vi "Read Size.vi"(8 "error in (no error)":errorcluster, 11 "Splitter in":refnum<class "Splitter.lvclass">) -> (0 "error out":errorcluster, 2 "Size":i32, 3 "Splitter out":refnum<class "Splitter.lvclass">)   [LabVIEW 2017, in "Splitter.lvclass"]
uses:
  Splitter.lvclass
  Splitter.lvclass/Splitter.ctl
  Low-Level VI Manipulation/Find Resource by Type (String).vi
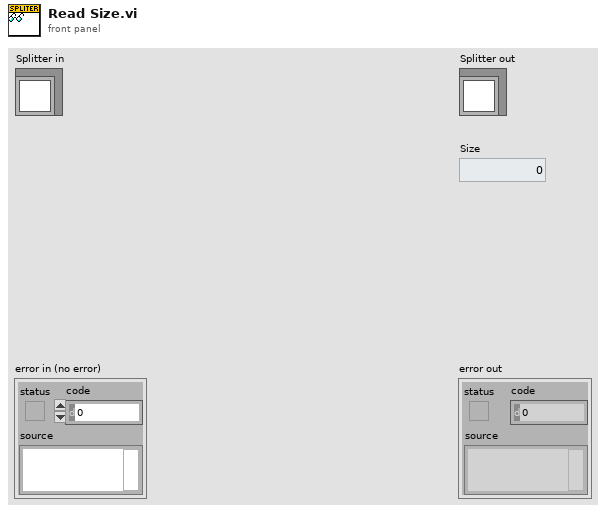
[diagram p1: front panel]
types:
  T1 = typedef "Resource Array.ctl" = T2[]
  T2 = typedef "Resource.ctl" = cluster{"type":u32, "id":i32, "name":string, "binary data":string}
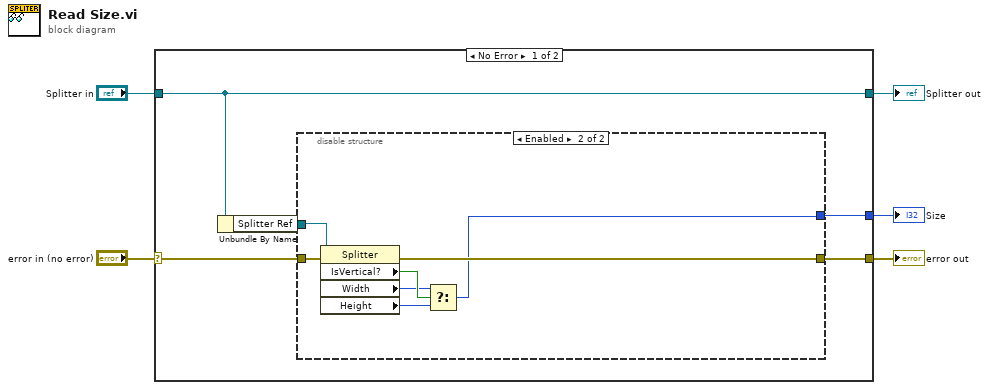
[diagram p0: block diagram]
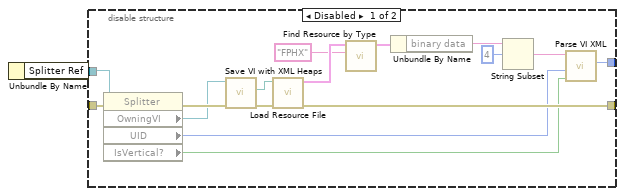
[diagram p2: hidden frame]
diagram:
  n1 = case shown="No Error" "error in (no error)" {
    selector: "error in (no error)" -> [w8 w35]
    tunnel: [w7 w35] -> w4
    tunnel: [w9 w36] -> w2
    tunnel: "Splitter in" -> [w9 w36]
    tunnel: [w6 _] -> w1
    frame No Error {
      n2 = disable-structure shown="Enabled" {
        disable-tunnel: w9 -> [w26 w34]
        disable-tunnel: w8 -> [w18 w33]
        disable-tunnel: [w17 w31] -> w7
        disable-tunnel: [w12 w27] -> w6
        frame Disabled {
          n3 = Unbundle By Name(w26) -> ("Splitter Ref"=w11:refnum<vi>)
          n4 = property class="Splitter"(reference=w11, error in=w18) -> (error out=w15:errorcluster, "OwningVI"=w10:refnum<vi>, "UID"=w14:i32, "IsVertical?"=w13:bool)  [unwired: 1 out]
          n5 = call "Save VI with XML Heaps.vi"("error in (no error)"=w15, "VI Refnum In"=w10) -> ("error out"=w19:errorcluster, "VI Path out"=w25:path)  [unwired: 7 in, 1 out]
          n6 = call "Load Resource File.vi"("error in (no error)"=w19, "Resource file"=w25) -> ("error out"=w17:errorcluster, "Resources"=w21:T1)  [unwired: 7 in, 1 out]
          n7 = call-poly "Find Resource by Type.vi"("Resource Type"="FPHX", "Resources"=w21) -> ("Resource"=w22:T2)  [unwired: 7 in, 2 out]
          n8 = Unbundle By Name(w22) -> ("binary data"=w23:string)
          n9 = String Subset(string=w23, offset (0)=4) -> (substring=w16:string)  [unwired: 1 in]
          n10 = call "Parse VI XML.vi"("Is Vertical?"=w13, "UID"=w14, "VI XML"=w16) -> ("Old Size"=w12:i32)  [unwired: 7 in, 1 out]
        }
        frame Enabled {
          n11 = Unbundle By Name(w34) -> ("Splitter Ref"=w32:refnum<vi>)
          n12 = property class="Splitter"(reference=w32, error in=w33) -> (error out=w31:errorcluster, "IsVertical?"=w30:bool, "Width"=w29:u32, "Height"=w28:u32)  [unwired: 1 out]
          n13 = Select(t=w29, s=w30, f=w28) -> (s? t:f=w27:u32)
        }
      }
    }
    frame Error {
    }
  }
  "error out" <- w4
  "Splitter out" <- w2
  "Size" <- w1
